vi "Send Get Notifiers Msg.vi"(8 "error in (no error)":errorcluster, 10 "Notifier of Notifiers":refnum<notifier>, 11 "Message Queue in":refnum<queue>) -> (0 "error out":errorcluster, 3 "Message Queue out":refnum<queue>)   [LabVIEW 2024, in "PID Loop.lvlib" / "Get Notifiers Msg.lvclass"]
uses:
  Get Notifiers Msg.lvclass
  src/Zero Timeout Message Handler/~Message/~Message.lvclass
  Get Notifiers Msg.lvclass/Get Notifiers Msg.ctl
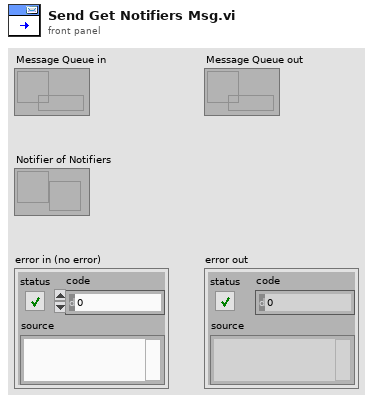
[diagram p1: front panel]
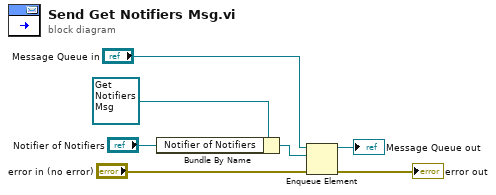
[diagram p0: block diagram]
diagram:
  n1 = Bundle By Name(cluster=refnum<class "Get Notifiers Msg.lvclass"> refnum ("PID Loop.lvlib:Get Notifiers Msg.lvclass"), "Notifier of Notifiers"="Notifier of Notifiers") -> (w5:refnum<class "Get Notifiers Msg.lvclass">)
  n2 = Enqueue Element(queue="Message Queue in", element=w5, error in (no error)="error in (no error)") -> (queue out=→"Message Queue out":refnum<queue>, error out=→"error out":errorcluster)  [unwired: 1 in, 1 out]
